vi "subjectType.vi"(8 "error in (no error)":errorcluster, 10 "file_type":T1, 11 "reference in":refnum<class "Subject Controller.lvclass">) -> (0 "error out":errorcluster, 3 "reference out":refnum<class "Subject Controller.lvclass">)   [LabVIEW 2015, in "Subject Controller.lvclass"]
uses:
  Subject Controller.lvclass
  APP/excelFile_class/fileType.ctl
  APP/excelFile_class/excelFile.lvclass
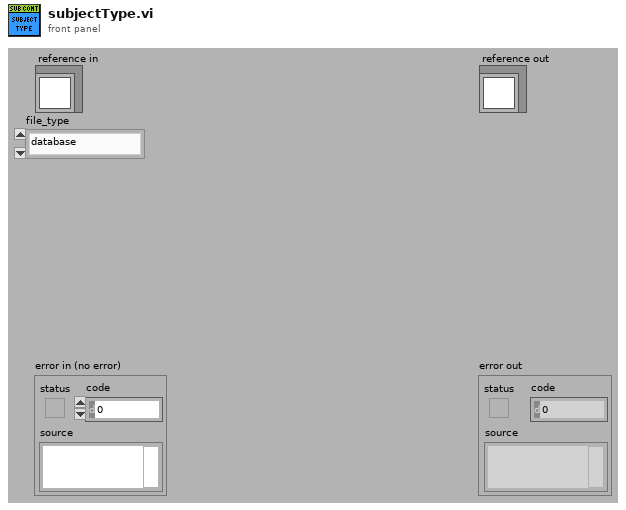
[diagram p1: front panel]
types:
  T1 = typedef "excelFile.lvclass/fileType.ctl" = enum16{"database", "CosmedTest PFTSUITE", "CosmedTest OMNIA"}
  T2 = typedef "Subject Controller.lvclass/ObjectAttributesRef.ctl" = refnum<data-value>
  T3 = typedef "Subject Controller.lvclass/ObjectAttributes.ctl" = cluster{"MyAttribute":dbl, "subject_controller_ref":refnum<class "Subject Controller.lvclass">, "file_controller_ref":refnum<class "File Controller.lvclass">, "subject_refs":refnum<class "subject.lvclass">[], "subjectIndex":i32, "file_type":T1}
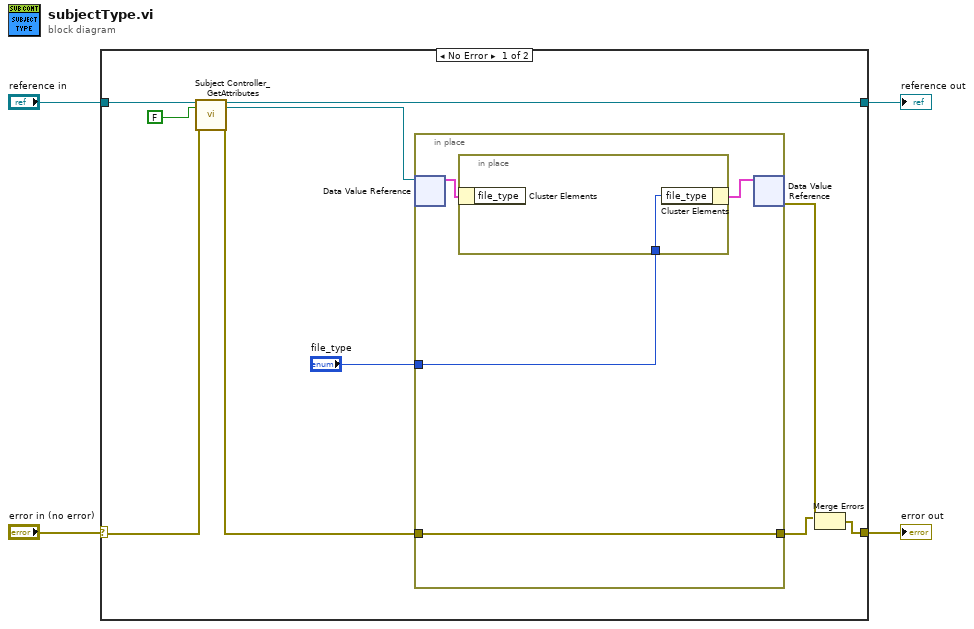
[diagram p0: block diagram]
diagram:
  n1 = case shown="No Error" "error in (no error)" {
    selector: "error in (no error)" -> [w10 w21]
    tunnel: [w6 w21] -> w3
    tunnel: [w8 w20] -> w1
    tunnel: "reference in" -> [w12 w20]
    frame No Error {
      n2 = call "Subject Controller_GetAttributes.vi"("reference in"=w12, "return data? (T)"=FALSE, "error in (no error)"=w10) -> ("reference out"=w8:refnum<class "Subject Controller.lvclass">, "attributes ref"=w7:T2, "error out"=w9:errorcluster)  [unwired: 13 in, 1 out]
      n3 = in-place {
        in-place-border: w9 -> [w16]
        in-place-border: [w16] -> w13
        in-place-border: "file_type" -> [w15]
        n4 = in-place-dvr #1(w7) -> (w17:T3)  [unwired: 1 out]
        n5 = in-place {
          in-place-border: w15 -> [w19]
          n6 = in-place-cluster #2(w17) -> ()  [unwired: 1 out]
          n7 = in-place-cluster #2("file_type"=w19) -> (w18:T3)
        }
        n8 = in-place-dvr #1(w18) -> (w14:errorcluster)  [unwired: 1 out]
      }
      n9 = Merge Errors(w13, w14) -> (w6:errorcluster)
    }
    frame Error {
    }
  }
  "error out" <- w3
  "reference out" <- w1
